vi "Camera Loop.vi"   [LabVIEW 2013]
uses:
  Camera Search State.ctl
  Robot Global Data.vi
  <vilib>/Rock Robotics/WPI/Gyro/WPI_GyroRefNum Registry Get.vi
  <vilib>/Rock Robotics/WPI/Gyro/WPI_GyroGetAngle.vi
types:
  T1 = typedef "Camera Search State.ctl" = enum16{"Manual", "Search Left", "Search Right", "Target Found", "Disabled", "Search Down", "Search Up"}
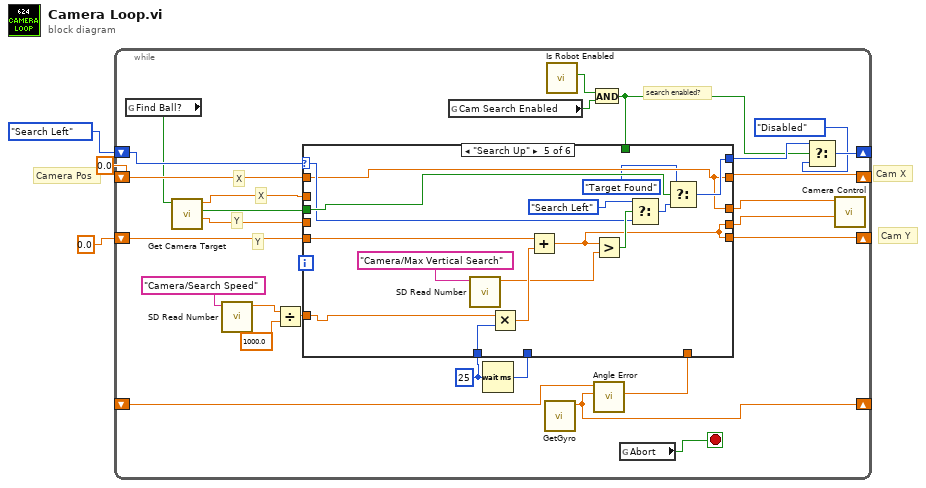
[diagram p0: block diagram]
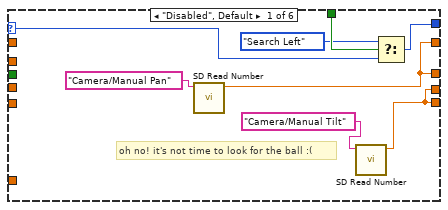
[diagram p2: hidden frame]
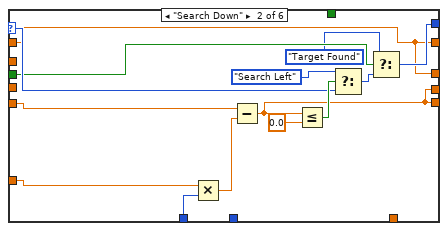
[diagram p3: hidden frame]
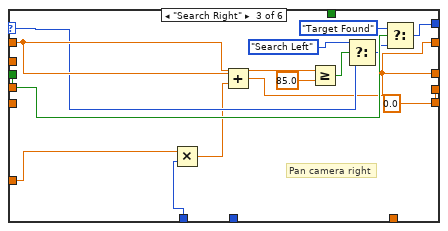
[diagram p4: hidden frame]
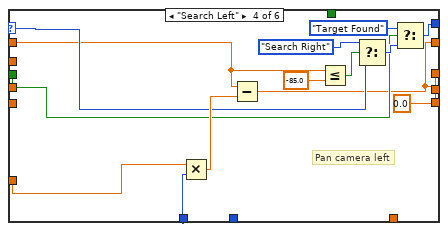
[diagram p5: hidden frame]
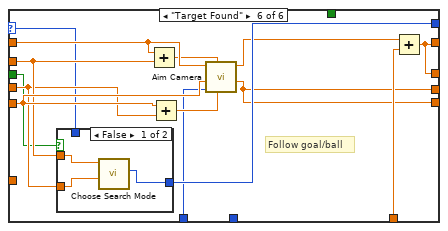
[diagram p6: hidden frame]
diagram:
  # "Camera Pos"
  # "Cam Y"
  # "Cam X"
  n1 = while {
    shift-right: [w21] -> _
    shift-left: 0.0 ("Current X") -> [w30]
    shift-right: [w29] -> _
    shift-left: 0.0 ("Current X") -> [w28]
    shift-right: [w6] -> _
    shift-left: _ -> [w5]
    shift-right: [w20] -> _
    shift-left: Camera_Search_State."Search Left" -> [w27]
    stop <- w4 stop-if-true
    w17 = u32 25 ("milliseconds to wait")
    # "Y"
    # "X"
    # "Y"
    # "X"
    # "search enabled?"
    n2 = global read "Robot Global Data.vi" "Find Ball?"() -> (w13:bool)
    n3 = call "Get Camera Target.vi"("Track Ball?"=w13) -> ("Camera Relative Y"=w16:dbl, "Found?"=w15:bool, "Camera Relative X"=w14:dbl)  [unwired: 8 in]
    n4 = call <vilib>:"SD Read Number.vi"("Name"="Camera/Search Speed") -> ("Numeric"=w25:dbl)  [unwired: 8 in, 2 out]
    n5 = Divide(x=w25, y=1000.0) -> (x/y=w23:dbl)
    n6 = global read "Robot Global Data.vi" "Cam Search Enabled"() -> (w12:bool)
    n7 = Wait (ms)(milliseconds to wait=w17) -> (millisecond timer value=w22:u32)
    n8 = call "GetGyro.vi"() -> ("Angle"=w6:dbl)  [unwired: 10 in, 1 out]
    n9 = call "Is Robot Enabled"() -> ("Enabled?"=w11:bool)  [unwired: 11 in]
    n10 = And(x=w11, y=w12) -> (x .and. y?=w18:bool)
    n11 = call "Angle Error.vi"("Angle"=w6, "Target Angle"=w5) -> ("Error"=w7:dbl)  [unwired: 9 in]
    n12 = case shown="\"Search Up\"" w27 {
      selector: w27 -> [w36 w44 w61 w73 w87 w103]
      tunnel: w30 -> [_ w42 w66 w72 w85 w109]
      tunnel: [w35 w42 w56 w71 w85 w104] -> w8
      tunnel: [w33 w49 w59 w69 w84 w100] -> w9
      tunnel: [w33 w49 w59 w69 w84 w100] -> w29
      tunnel: w28 -> [_ w45 _ _ w89 w108]
      tunnel: w17 -> [_ w46 w57 w76 w83 w96]
      tunnel: w14 -> [_ _ _ _ _ w107]
      tunnel: w16 -> [_ _ _ _ _ w106]
      tunnel: [w35 w42 w56 w71 w85 w104] -> w21
      tunnel: [w38 w52 w60 w70 w86 w101] -> w19
      tunnel: w15 -> [_ w43 w64 w74 w88 w102]
      tunnel: w23 -> [_ w47 w58 w75 w90 _]
      tunnel: w22 -> [_ _ _ _ _ _]
      tunnel: w7 -> [_ _ _ _ _ w105]
      tunnel: w18 -> [w37 _ _ _ _ _]
      frame "Disabled", Default {
        # "oh no! it's not time to look for the ball :("
        n13 = call <vilib>:"SD Read Number.vi"("Name"="Camera/Manual Pan") -> ("Numeric"=w35:dbl)  [unwired: 8 in, 2 out]
        n14 = call <vilib>:"SD Read Number.vi"("Name"="Camera/Manual Tilt") -> ("Numeric"=w33:dbl)  [unwired: 8 in, 2 out]
        n15 = Select(t=Camera_Search_State."Search Left", s=w37, f=w36) -> (s? t:f=w38:T1)
      }
      frame "Search Down" {
        n16 = Multiply(x=w47, y=w46) -> (x*y=w48:dbl)
        n17 = Subtract(x=w45, y=w48) -> (x-y=w49:dbl)
        n18 = Less Or Equal?(x=w49, y=0.0) -> (x <= y?=w50:bool)
        n19 = Select(t=Camera_Search_State."Search Left", s=w50, f=w44) -> (s? t:f=w51:T1)
        n20 = Select(t=Camera_Search_State."Target Found", s=w43, f=w51) -> (s? t:f=w52:T1)
      }
      frame "Search Right" {
        w59 = 0.0
        # "Pan camera right"
        n21 = Multiply(x=w58, y=w57) -> (x*y=w55:dbl)
        n22 = Add(x=w66, y=w55) -> (x+y=w56:dbl)
        n23 = Greater Or Equal?(x=w66, y=85.0) -> (x >= y?=w63:bool)
        n24 = Select(t=Camera_Search_State."Search Left", s=w63, f=w61) -> (s? t:f=w62:T1)
        n25 = Select(t=Camera_Search_State."Target Found", s=w64, f=w62) -> (s? t:f=w60:T1)
      }
      frame "Search Left" {
        w69 = 0.0
        # "Pan camera left"
        n26 = Multiply(x=w75, y=w76) -> (x*y=w80:dbl)
        n27 = Subtract(x=w72, y=w80) -> (x-y=w71:dbl)
        n28 = Less Or Equal?(x=w72, y=-85.0) -> (x <= y?=w78:bool)
        n29 = Select(t=Camera_Search_State."Search Right", s=w78, f=w73) -> (s? t:f=w77:T1)
        n30 = Select(t=Camera_Search_State."Target Found", s=w74, f=w77) -> (s? t:f=w70:T1)
      }
      frame "Search Up" {
        n31 = call <vilib>:"SD Read Number.vi"("Name"="Camera/Max Vertical Search") -> ("Numeric"=w92:dbl)  [unwired: 8 in, 2 out]
        n32 = Multiply(x=w90, y=w83) -> (x*y=w93:dbl)
        n33 = Add(x=w89, y=w93) -> (x+y=w84:dbl)
        n34 = Greater?(x=w84, y=w92) -> (0:w94:bool)
        n35 = Select(t=Camera_Search_State."Search Left", s=w94, f=w87) -> (s? t:f=w95:T1)
        n36 = Select(t=Camera_Search_State."Target Found", s=w88, f=w95) -> (s? t:f=w86:T1)
      }
      frame "Target Found" {
        # "Follow goal/ball"
        n37 = case shown="False" w102 {
          tunnel: w103 -> [_ w113]
          tunnel: [w112 w113] -> w101
          tunnel: w107 -> [w110 _]
          tunnel: w106 -> [w111 _]
          frame False {
            n38 = call "Choose Search Mode.vi"("Last Cam-Relative Y"=w111, "Last Cam-Relative X"=w110) -> ("Search Dir"=w112:T1)  [unwired: 9 in]
          }
          frame True {
          }
        }
        n39 = Add(x=w109, y=w107) -> (x+y=w97:dbl)
        n40 = Add(x=w108, y=w106) -> (x+y=w98:dbl)
        n41 = call "Aim Camera.vi"("Target Y"=w98, "Target X"=w97, "time difference (ms)"=w96, "Old Y"=w108, "Old X"=w109) -> ("Current Y"=w100:dbl, "Current X"=w99:dbl)  [unwired: 3 in, 2 out]
        n42 = Add(x=w99, y=w105) -> (x+y=w104:dbl)
      }
    }
    n43 = global read "Robot Global Data.vi" "Abort"() -> (w4:bool)
    n44 = Select(t=w19, s=w18, f=Camera_Search_State."Disabled") -> (s? t:f=w20:T1)
    n45 = call "Camera Control.vi"("Y Degrees"=w9, "X  Degrees"=w8) -> ()  [unwired: 10 in]
  }
